vi "PWM Manual.vi"() -> ()   [LabVIEW 2016]
panel:
  in  "Valor Constante":dbl(knob) scale=0.0..100.0
  in  "Desfase":dbl(knob) scale=-100.0..100.0
  in  "Muestras":i32(knob) scale=100.0..1000.0
  out "Waveform Graph":dbl[][](graph)
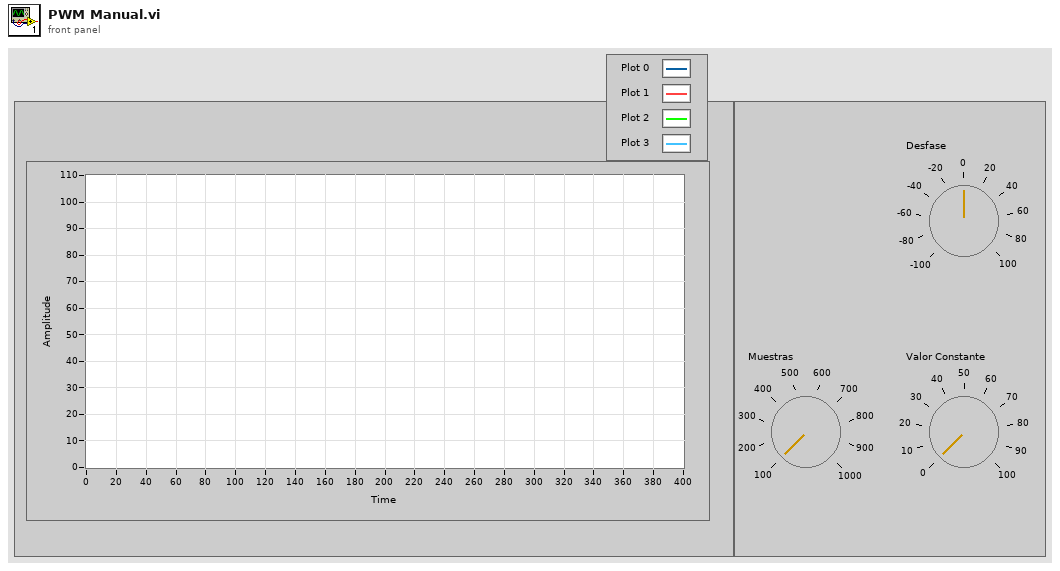
[diagram p1: front panel]
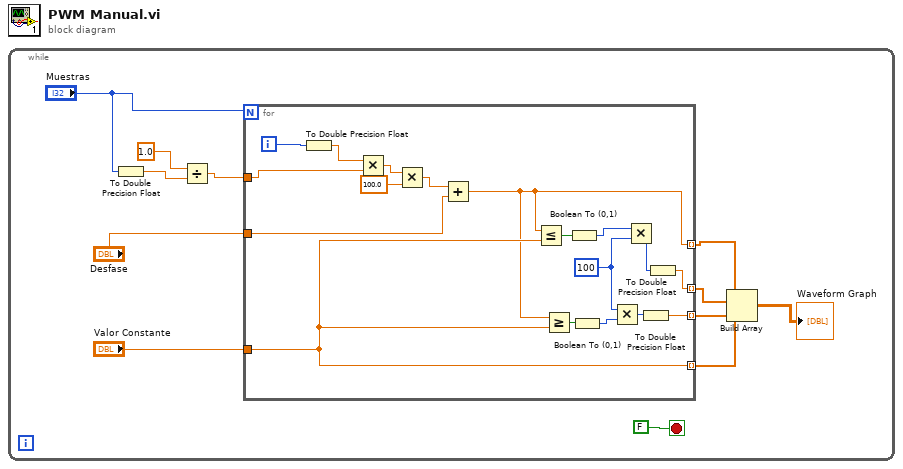
[diagram p0: block diagram]
diagram:
  n1 = while {
    stop <- FALSE stop-if-true
    n2 = To Double Precision Float(number="Muestras") -> (double precision float=w7:dbl)
    n3 = Divide(x=1.0, y=w7) -> (x/y=w5:dbl)
    n4 = for {
      N: "Muestras" -> [_]
      tunnel: "Valor Constante" -> [w21]
      tunnel: [w21] -> w4 mode=indexing
      tunnel: [w13] -> w10 mode=indexing
      tunnel: w5 -> [w30]
      tunnel: [w22] -> w2 mode=indexing
      tunnel: [w16] -> w3 mode=indexing
      tunnel: "Desfase" -> [w14]
      i -> [w29]
      w18 = i16 100 ("y")
      n5 = To Double Precision Float(number=w29) -> (double precision float=w28:dbl)
      n6 = Multiply(x=w28, y=w30) -> (x*y=w27:dbl)
      n7 = Multiply(x=w27, y=100.0) -> (x*y=w15:dbl)
      n8 = Add(x=w15, y=w14) -> (x+y=w13:dbl)
      n9 = Less Or Equal?(x=w13, y=w21) -> (x <= y?=w25:bool)
      n10 = Greater Or Equal?(x=w13, y=w21) -> (x >= y?=w20:bool)
      n11 = Boolean To (0,1)(Boolean=w25) -> (0, 1=w24:i16)
      n12 = Boolean To (0,1)(Boolean=w20) -> (0, 1=w19:i16)
      n13 = Multiply(x=w18, y=w19) -> (x*y=w17:i16)
      n14 = Multiply(x=w24, y=w18) -> (x*y=w23:i16)
      n15 = To Double Precision Float(number=w17) -> (double precision float=w16:dbl)
      n16 = To Double Precision Float(number=w23) -> (double precision float=w22:dbl)
    }
    n17 = Build Array(w10, w2, w3, w4) -> (→"Waveform Graph":dbl[][])
  }
